vi "ConfigAcq.vi"(8 "error in (no error)":errorcluster, 11 "Agilent_3458A in":refnum<class "Agilent_3458A.lvclass">) -> (0 "error out":errorcluster, 3 "Agilent_3458A out":refnum<class "Agilent_3458A.lvclass">)   [LabVIEW 2018, in "DigitizerPlugins.lvlib" / "Agilent_3458A.lvclass"]
uses:
  Agilent_3458A.lvclass
  Y:/Projects/PMUCal/Modules/Digitizer/DigitizerPlugins/DigitizerBaseClass/DigitizerBase.lvclass
  DigitizerBaseClass/DigitizerBase.lvclass/DigitizerBase.ctl
  DigitizerBaseClass/Accessors/Read InstRef.vi
  DigitizerBaseClass/Accessors/Read Acquisition.vi
  <instrlib>/Agilent 3458/Agilent 3458.lvlib
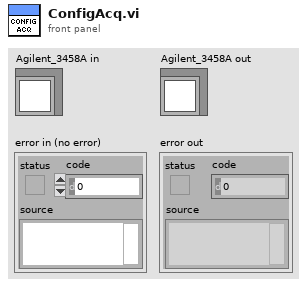
[diagram p1: front panel]
types:
  T1 = typedef "DigitizerPlugins.lvlib/DigitizerBase.lvclass/Acquisition.ctl" = cluster{"SampleRate":dbl, "RecordSize":i32, "NumRecords":i32, "SampleMode":i32, "Timeout (ms)":i32}
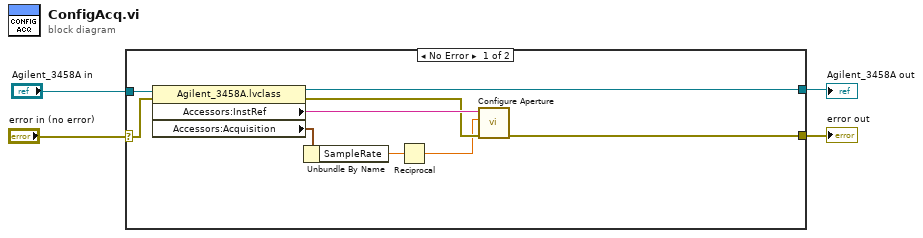
[diagram p0: block diagram]
diagram:
  n1 = case shown="No Error" "error in (no error)" {
    selector: "error in (no error)" -> [w12 w15]
    tunnel: "Agilent_3458A in" -> [w13 w14]
    tunnel: [w9 w14] -> w2
    tunnel: [w5 w15] -> w1
    frame No Error {
      n2 = property class="Agilent_3458A.lvclass"(reference=w13, error in=w12) -> (reference out=w9:refnum<class "Agilent_3458A.lvclass">, error out=w8:errorcluster, "Accessors:InstRef"=w11:string, "Accessors:Acquisition"=w10:T1)
      n3 = Unbundle By Name(w10) -> ("SampleRate"=w7:dbl)
      n4 = Reciprocal(x=w7) -> (1/x=w6:dbl)
      n5 = call <instrlib>:"Configure Aperture.vi"("error in (no error)"=w8, "Aperture Time (5.00E-9 s)"=w6, "VISA resource name"=w11) -> ("error out"=w5:errorcluster)  [unwired: 7 in, 1 out]
    }
    frame Error {
    }
  }
  "error out" <- w1
  "Agilent_3458A out" <- w2
